vi "Write Port.vi"(8 "error in":errorcluster, 10 "port":u16, 11 "TCP master in":refnum<class "TCP Interface.lvclass">) -> (0 "error out":errorcluster, 3 "TCP master out":refnum<class "TCP Interface.lvclass">)   [LabVIEW 2021, in "TCP Interface.lvclass"]
doc: "Property accessor for the TCP port."
uses:
  TCP Interface.lvclass
  TCP Interface.lvclass/TCP Interface.ctl
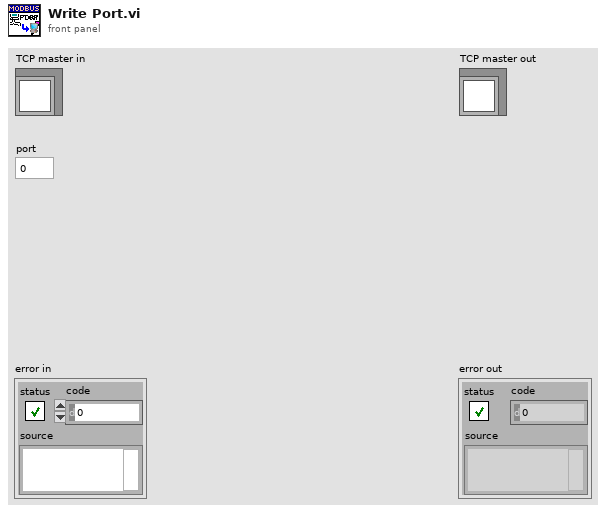
[diagram p1: front panel]
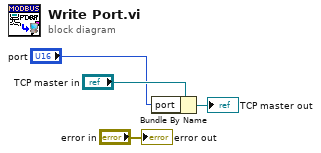
[diagram p0: block diagram]
diagram:
  n1 = Bundle By Name(cluster="TCP master in", "port"="port") -> (→"TCP master out":refnum<class "TCP Interface.lvclass">)
  "error out" <- "error in"
